vi "HumanElevatorWristTeleop.vi"(0 "CmdElevRestWristRest":bool, 4 "CmdElevWristSource":bool, 5 "CmdElevAlgae2WristFlat":bool, 6 "CmdElevWristCancel":bool, 7 "CmdElevAlgae1WristFlat":bool, 8 "CmdElevL4WristSlant":bool, 9 "CmdElevL3WristFlat":bool, 10 "CmdElevL2WristFlat":bool, 11 "CmdElevL1WristFlat":bool) -> ()   [LabVIEW 2023]
uses:
  <vilib>/Rock Robotics/WPI/ThirdParty/JAS_Junk/TrajLib/VI/DigSeqLogic_Edge_On.vi
  Elevator/ElevatorBargeSendCmd.vi
  Elevator/ElevatorFloorSendCmd.vi
  Elevator/ElevSendDecCmd.vi
  Elevator/ElevSendIncCmd.vi
  Elevator/ElevatorCancelCmd.vi
  Elevator/ElevatorL4SendCmd.vi
  Elevator/ElevatorAlgae1SendCmd.vi
  Elevator/ElevatorL3SendCmd.vi
  Elevator/ElevatorAlgae2SendCmd.vi
  Elevator/ElevatorSourceSendCmd.vi
  Elevator/ElevatorL2SendCmd.vi
  Elevator/ElevatorL1SendCmd.vi
  Elevator/ElevatorRestSendCmd.vi
panel:
  in  "CmdElevSrc3":bool
  in  "CmdElevFloorWristFlat":bool
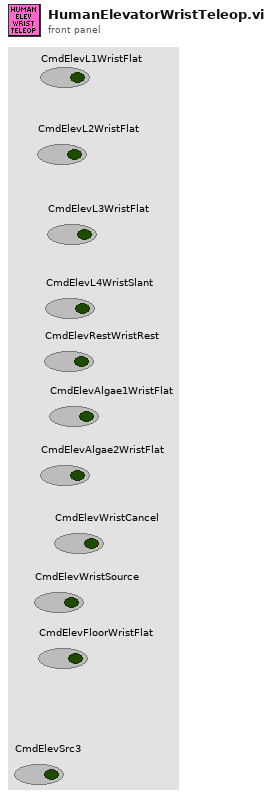
[diagram p1: front panel]
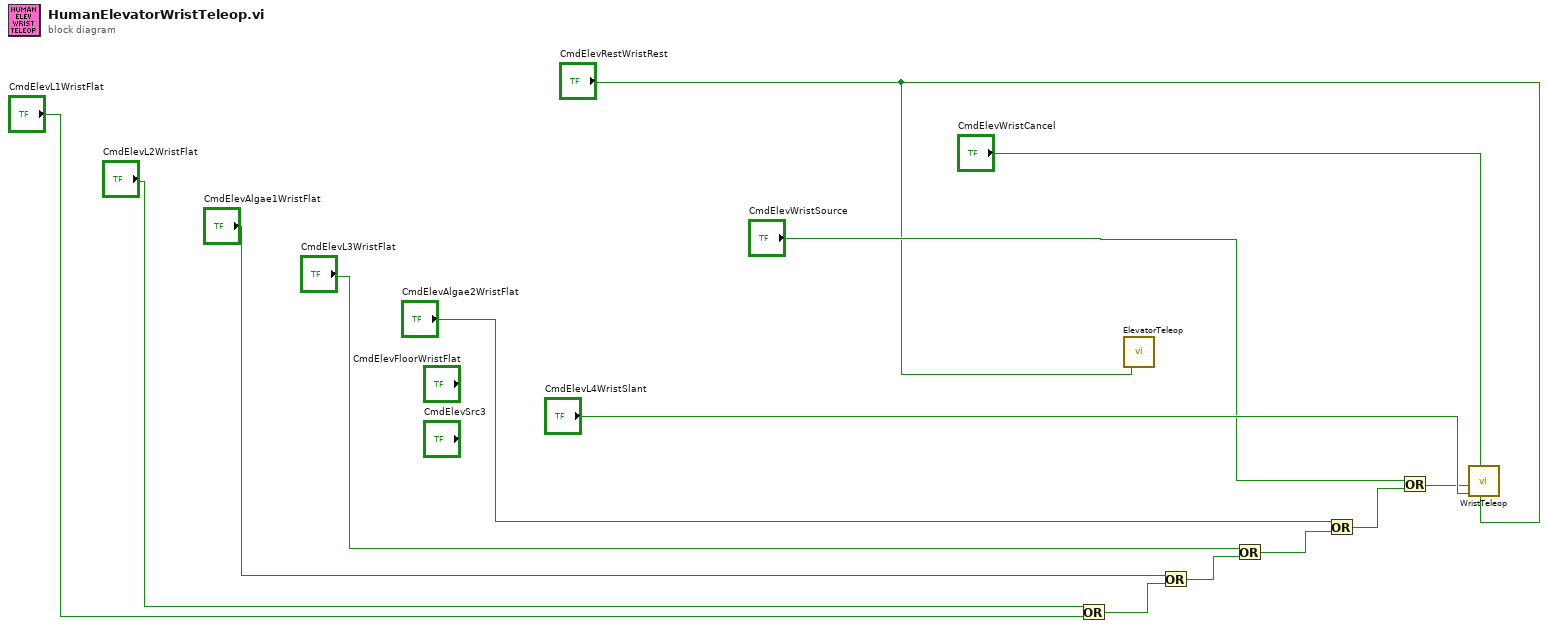
[diagram p0: block diagram]
diagram:
  n1 = Or(x="CmdElevL2WristFlat", y="CmdElevL1WristFlat") -> (x .or. y?=w8:bool)
  n2 = call "ElevatorTeleop.vi"("CmdElevRest"="CmdElevRestWristRest") -> ()  [unwired: 19 in]
  n3 = Or(x="CmdElevAlgae1WristFlat", y=w8) -> (x .or. y?=w10:bool)
  n4 = Or(x="CmdElevL3WristFlat", y=w10) -> (x .or. y?=w12:bool)
  n5 = Or(x="CmdElevAlgae2WristFlat", y=w12) -> (x .or. y?=w4:bool)
  n6 = Or(x="CmdElevWristSource", y=w4) -> (x .or. y?=w3:bool)
  n7 = call "WristTeleop.vi"("Rest"="CmdElevRestWristRest", "Cancel"="CmdElevWristCancel", "Slant"="CmdElevL4WristSlant", "Flat"=w3) -> ()  [unwired: 8 in]
